vi "Version_4.9_8_on-chip_valves_for25ulSyringe_withModfied_Plunging.vi"() -> ()   [LabVIEW 2020] (continued)
                            n2712 = local write "Valve V2 Open"(FALSE ("Valve V2 Open")) -> ()
                            n2713 = local write "Valve V3 Open"(FALSE ("Valve V3 Open")) -> ()
                            n2714 = local write "Valve V4 Open"(TRUE ("Valve V4 Open")) -> ()
                            n2715 = call "PortChanger_Valve (SubVI).vi"("Port Number"=w3158, "VISA Refnum in"=w3159) -> ()  [unwired: 10 in]
                            n2716 = local write "Valve V5 Open"(TRUE ("Valve V5 Open")) -> ()
                            n2717 = local write "Valve V6 Open"(TRUE ("Valve V6 Open")) -> ()
                            n2718 = local write "Valve V7 Open"(FALSE ("Valve V7 Open")) -> ()
                          }
                          frame #3 {
                            n2719 = local read "Apparent Volume\nof Syringe"() -> (w3164:dbl)
                            n2720 = local read "Sample Volume \nto be Pumped"() -> (w3167:dbl)
                            n2721 = Quotient & Remainder(x=w3167, y=w3164) -> (x-y*floor(x/y)=w3165:dbl, floor(x/y)=w3166:dbl)
                            n2722 = for {
                              N: w3166 -> [_]
                              n2723 = stacked-sequence {
                                frame #0 {
                                n2724 = local read "Sample PickUp \nFlow Rate (ul/min)"() -> (w3170:dbl)
                                n2725 = local read "Sample Pumping\nResolution"() -> (w3169:T2)
                                n2726 = local read "VISA Refnum in\nfor Pump"() -> (w3172:refnum<visa-resource-name>)
                                n2727 = local read "Apparent Volume\nof Syringe"() -> (w3168:dbl)
                                n2728 = local read "Volume of Syringe"() -> (w3171:dbl)
                                n2729 = call "RPickUp(SubVI).vi"("Volume to be picked up"=w3168, "Volume of Syringe"=w3171, "Resolution of PickUP"=w3169, "PickUp Flow Rate (ul/min)"=w3170, "VISA Refnum in"=w3172) -> ()  [unwired: 6 in, 1 out]
                                }
                                frame #1 {
                                n2730 = local read "Stopper that ends \nthe main loops"() -> (w3173:bool)
                                n2731 = local read "VISA Refnum in\nfor Pump"() -> (w3174:refnum<visa-resource-name>)
                                n2732 = case shown="True" w3173 {
                                frame False {
                                }
                                frame True {
                                n2733 = local read "VISA Refnum in\nfor Pump"() -> (w3175:refnum<visa-resource-name>)
                                n2734 = call "HardStopCurrentProcess (SubVI).vi"("VISA Refnum in"=w3175) -> ()  [unwired: 11 in]
                                }
                                }
                                n2735 = call "ProcessCompletionWaiter (SubVI).vi"("VISA Refnum in"=w3174) -> ()  [unwired: 11 in]
                                }
                                frame #2 {
                                # "Reads the initial Plunger Position for computing the volume dispensed"
                                n2736 = local read "VISA Refnum in\nfor Pump"() -> (w3177:refnum<visa-resource-name>)
                                n2737 = call "AbsolutePlungerPosition (SubVI).vi"("VISA Refnum in"=w3177) -> ("Plunger Position"=w3176:i32)  [unwired: 10 in]
                                n2738 = local write "Initial Plunger Position"(w3176) -> ()
                                }
                                frame #3 {
                                # "Switch to Port-2"
                                # "Port-2 of the pump is conncted to column-1 of chip"
                                n2739 = local read "VISA Refnum in\nfor Pump"() -> (w3179:refnum<visa-resource-name>)
                                n2740 = call "PortChanger (SubVI).vi"("Port Number"="10", "VISA Refnum in"=w3179) -> ()  [unwired: 10 in]
                                }
                                frame #4 {
                                n2741 = local read "Stopper that ends \nthe main loops"() -> (w3180:bool)
                                n2742 = local read "VISA Refnum in\nfor Pump"() -> (w3181:refnum<visa-resource-name>)
                                n2743 = case shown="True" w3180 {
                                frame False {
                                }
                                frame True {
                                n2744 = local read "VISA Refnum in\nfor Pump"() -> (w3182:refnum<visa-resource-name>)
                                n2745 = call "HardStopCurrentProcess (SubVI).vi"("VISA Refnum in"=w3182) -> ()  [unwired: 11 in]
                                }
                                }
                                n2746 = call "ProcessCompletionWaiter (SubVI).vi"("VISA Refnum in"=w3181) -> ()  [unwired: 11 in]
                                }
                                frame #5 {
                                # "Keeps the AMF valve after column-1 open and valve after column-2 closed"
                                n2747 = local read "Sample Dispense\nFlow Rate (ul/min)"() -> (w3186:dbl)
                                n2748 = local read "Sample Pumping\nResolution"() -> (w3185:T2)
                                n2749 = local read "VISA Refnum in\nfor Pump"() -> (w3188:refnum<visa-resource-name>)
                                n2750 = local write "Pause Data Collection"(FALSE ("Pause Data Collection")) -> ()
                                n2751 = local read "Volume of Syringe"() -> (w3187:dbl)
                                n2752 = call "GoToAbsolutePosition(SubVI).vi"("Absolute Volume Position in Syringe (in ul)"=0.0 ("Volume to be Dispensed"), "Volume of Syringe"=w3187, "Resolution of Pumping"=w3185, "Flow Rate (ul/min)"=w3186, "VISA Refnum in"=w3188) -> ()  [unwired: 6 in, 1 out]
                                }
                                frame #6 {
                                n2753 = local read "Sample Pumping\nResolution"() -> (w3190:T2)
                                n2754 = local read "VISA Refnum in\nfor Pump"() -> (w3192:refnum<visa-resource-name>)
                                n2755 = local read "Initial Plunger Position"() -> (w3191:dbl)
                                n2756 = local read "Volume of Syringe"() -> (w3189:dbl)
                                n2757 = while {
                                tunnel: w3191 -> [w3199]
                                tunnel: w3192 -> [w3198]
                                tunnel: w3190 -> [w3197]
                                tunnel: w3189 -> [w3196]
                                stop <- w3194 stop-if-true
                                n2758 = stacked-sequence {
                                tunnel: w3199 -> [w3206 _]
                                tunnel: w3198 -> [w3205 w3226]
                                tunnel: w3197 -> [w3204 _]
                                tunnel: w3196 -> [w3203 _]
                                tunnel: [_ w3224] -> w3194
                                frame #0 {
                                n2759 = call "AbsolutePlungerPosition (SubVI).vi"("VISA Refnum in"=w3205) -> ("Plunger Position"=w3202:i32)  [unwired: 10 in]
                                n2760 = case shown="\"Standard Pumping\", Default" w3204 {
                                tunnel: w3206 -> [w3211 w3220]
                                tunnel: w3202 -> [w3212 w3219]
                                tunnel: [w3210 w3217] -> w3201
                                tunnel: w3203 -> [w3209 w3218]
                                frame "Standard Pumping", Default {
                                n2761 = Subtract(x=w3211, y=w3212) -> (x-y=w3208:dbl)
                                n2762 = Absolute Value(x=w3208) -> (abs(x)=w3207:dbl)
                                n2763 = Multiply(x=w3207, y=w3209) -> (x*y=w3214:dbl)
                                n2764 = Divide(x=w3214, y=3000.0) -> (x/y=w3210:dbl)
                                }
                                frame "High Resolution Pumping" {
                                n2765 = Subtract(x=w3220, y=w3219) -> (x-y=w3216:dbl)
                                n2766 = Absolute Value(x=w3216) -> (abs(x)=w3215:dbl)
                                n2767 = Multiply(x=w3215, y=w3218) -> (x*y=w3222:dbl)
                                n2768 = Divide(x=w3222, y=24000.0) -> (x/y=w3217:dbl)
                                }
                                }
                                n2769 = local write "Volume being Injected \nin this process"(w3201) -> ()
                                }
                                frame #1 {
                                n2770 = call "LSPOneStatus (SubVI).vi"("VISA Refnum in"=w3226) -> ("read buffer"=w3228:string)  [unwired: 10 in]
                                n2771 = call <vilib>:"Trim Whitespace.vi"("string"=w3228) -> ("trimmed string"=w3227:string)  [unwired: 1 in]
                                n2772 = local read "Stopper that ends \nthe main loops"() -> (w3223:bool)
                                n2773 = Equal?(x=w3227, y="/0`\u0003") -> (x = y?=w3225:bool)
                                n2774 = Or(x=w3225, y=w3223) -> (x .or. y?=w3224:bool)
                                }
                                }
                                n2775 = Wait (ms)(milliseconds to wait=u32 100) -> ()  [unwired: 1 out]
                                n2776 = local read "Stopper that ends \nthe main loops"() -> (w3193:bool)
                                n2777 = case shown="True" w3193 {
                                frame False {
                                }
                                frame True {
                                n2778 = local read "VISA Refnum in\nfor Pump"() -> (w3200:refnum<visa-resource-name>)
                                n2779 = call "HardStopCurrentProcess (SubVI).vi"("VISA Refnum in"=w3200) -> ()  [unwired: 11 in]
                                }
                                }
                                }
                                }
                                frame #7 {
                                # "Chnage the pump port back to Sample"
                                n2780 = local read "VISA Refnum in\nfor Pump"() -> (w3231:refnum<visa-resource-name>)
                                n2781 = local read "Port for \nSample"() -> (w3230:string)
                                n2782 = local write "Pause Data Collection"(TRUE ("Pause Data Collection")) -> ()
                                n2783 = Wait (ms)(milliseconds to wait=u32 500) -> ()  [unwired: 1 out]
                                n2784 = call "PortChanger (SubVI).vi"("Port Number"=w3230, "VISA Refnum in"=w3231) -> ()  [unwired: 10 in]
                                }
                                frame #8 {
                                n2785 = local read "VISA Refnum in\nfor Pump"() -> (w3234:refnum<visa-resource-name>)
                                n2786 = local write "Volume being Injected \nin this process"(0.0 ("Volume being Injected \nin this process")) -> ()
                                n2787 = call "ProcessCompletionWaiter (SubVI).vi"("VISA Refnum in"=w3234) -> ()  [unwired: 11 in]
                                }
                              }
                            }
                            n2788 = local write "Reminder of the \nVolume to be \nPumped"(w3165) -> ()
                          }
                          frame #4 {
                            n2789 = stacked-sequence {
                              frame #0 {
                                n2790 = local read "Sample PickUp \nFlow Rate (ul/min)"() -> (w3238:dbl)
                                n2791 = local read "Sample Pumping\nResolution"() -> (w3237:T2)
                                n2792 = local read "VISA Refnum in\nfor Pump"() -> (w3240:refnum<visa-resource-name>)
                                n2793 = local read "Reminder of the \nVolume to be \nPumped"() -> (w3236:dbl)
                                n2794 = local read "Volume of Syringe"() -> (w3239:dbl)
                                n2795 = call "RPickUp(SubVI).vi"("Volume to be picked up"=w3236, "Volume of Syringe"=w3239, "Resolution of PickUP"=w3237, "PickUp Flow Rate (ul/min)"=w3238, "VISA Refnum in"=w3240) -> ()  [unwired: 6 in, 1 out]
                              }
                              frame #1 {
                                n2796 = local read "Stopper that ends \nthe main loops"() -> (w3241:bool)
                                n2797 = local read "VISA Refnum in\nfor Pump"() -> (w3242:refnum<visa-resource-name>)
                                n2798 = case shown="True" w3241 {
                                frame False {
                                }
                                frame True {
                                n2799 = local read "VISA Refnum in\nfor Pump"() -> (w3243:refnum<visa-resource-name>)
                                n2800 = call "HardStopCurrentProcess (SubVI).vi"("VISA Refnum in"=w3243) -> ()  [unwired: 11 in]
                                }
                                }
                                n2801 = call "ProcessCompletionWaiter (SubVI).vi"("VISA Refnum in"=w3242) -> ()  [unwired: 11 in]
                              }
                              frame #2 {
                                # "Reads the initial Plunger Position for computing the volume dispensed"
                                n2802 = local read "VISA Refnum in\nfor Pump"() -> (w3245:refnum<visa-resource-name>)
                                n2803 = call "AbsolutePlungerPosition (SubVI).vi"("VISA Refnum in"=w3245) -> ("Plunger Position"=w3244:i32)  [unwired: 10 in]
                                n2804 = local write "Initial Plunger Position"(w3244) -> ()
                              }
                              frame #3 {
                                # "Switch to Port-2"
                                # "Port-2 of the pump is conncted to column-1 of chip"
                                n2805 = local read "VISA Refnum in\nfor Pump"() -> (w3247:refnum<visa-resource-name>)
                                n2806 = call "PortChanger (SubVI).vi"("Port Number"="10", "VISA Refnum in"=w3247) -> ()  [unwired: 10 in]
                              }
                              frame #4 {
                                n2807 = local read "Stopper that ends \nthe main loops"() -> (w3248:bool)
                                n2808 = local read "VISA Refnum in\nfor Pump"() -> (w3249:refnum<visa-resource-name>)
                                n2809 = case shown="True" w3248 {
                                frame False {
                                }
                                frame True {
                                n2810 = local read "VISA Refnum in\nfor Pump"() -> (w3250:refnum<visa-resource-name>)
                                n2811 = call "HardStopCurrentProcess (SubVI).vi"("VISA Refnum in"=w3250) -> ()  [unwired: 11 in]
                                }
                                }
                                n2812 = call "ProcessCompletionWaiter (SubVI).vi"("VISA Refnum in"=w3249) -> ()  [unwired: 11 in]
                              }
                              frame #5 {
                                # "Keeps the AMF valve after column-1 open and valve after column-2 closed"
                                n2813 = local read "Sample Dispense\nFlow Rate (ul/min)"() -> (w3254:dbl)
                                n2814 = local read "Sample Pumping\nResolution"() -> (w3253:T2)
                                n2815 = local read "VISA Refnum in\nfor Pump"() -> (w3256:refnum<visa-resource-name>)
                                n2816 = local write "Pause Data Collection"(FALSE ("Pause Data Collection")) -> ()
                                n2817 = local read "Volume of Syringe"() -> (w3255:dbl)
                                n2818 = call "GoToAbsolutePosition(SubVI).vi"("Absolute Volume Position in Syringe (in ul)"=0.0 ("Volume to be Dispensed"), "Volume of Syringe"=w3255, "Resolution of Pumping"=w3253, "Flow Rate (ul/min)"=w3254, "VISA Refnum in"=w3256) -> ()  [unwired: 6 in, 1 out]
                              }
                              frame #6 {
                                n2819 = local read "Sample Pumping\nResolution"() -> (w3258:T2)
                                n2820 = local read "VISA Refnum in\nfor Pump"() -> (w3260:refnum<visa-resource-name>)
                                n2821 = local read "Initial Plunger Position"() -> (w3259:dbl)
                                n2822 = local read "Volume of Syringe"() -> (w3257:dbl)
                                n2823 = while {
                                tunnel: w3259 -> [w3267]
                                tunnel: w3260 -> [w3266]
                                tunnel: w3258 -> [w3265]
                                tunnel: w3257 -> [w3264]
                                stop <- w3262 stop-if-true
                                n2824 = stacked-sequence {
                                tunnel: w3267 -> [w3274 _]
                                tunnel: w3266 -> [w3273 w3294]
                                tunnel: w3265 -> [w3272 _]
                                tunnel: w3264 -> [w3271 _]
                                tunnel: [_ w3292] -> w3262
                                frame #0 {
                                n2825 = call "AbsolutePlungerPosition (SubVI).vi"("VISA Refnum in"=w3273) -> ("Plunger Position"=w3270:i32)  [unwired: 10 in]
                                n2826 = case shown="\"Standard Pumping\", Default" w3272 {
                                tunnel: w3274 -> [w3279 w3288]
                                tunnel: w3270 -> [w3280 w3287]
                                tunnel: [w3278 w3285] -> w3269
                                tunnel: w3271 -> [w3277 w3286]
                                frame "Standard Pumping", Default {
                                n2827 = Subtract(x=w3279, y=w3280) -> (x-y=w3276:dbl)
                                n2828 = Absolute Value(x=w3276) -> (abs(x)=w3275:dbl)
                                n2829 = Multiply(x=w3275, y=w3277) -> (x*y=w3282:dbl)
                                n2830 = Divide(x=w3282, y=3000.0) -> (x/y=w3278:dbl)
                                }
                                frame "High Resolution Pumping" {
                                n2831 = Subtract(x=w3288, y=w3287) -> (x-y=w3284:dbl)
                                n2832 = Absolute Value(x=w3284) -> (abs(x)=w3283:dbl)
                                n2833 = Multiply(x=w3283, y=w3286) -> (x*y=w3290:dbl)
                                n2834 = Divide(x=w3290, y=24000.0) -> (x/y=w3285:dbl)
                                }
                                }
                                n2835 = local write "Volume being Injected \nin this process"(w3269) -> ()
                                }
                                frame #1 {
                                n2836 = call "LSPOneStatus (SubVI).vi"("VISA Refnum in"=w3294) -> ("read buffer"=w3296:string)  [unwired: 10 in]
                                n2837 = call <vilib>:"Trim Whitespace.vi"("string"=w3296) -> ("trimmed string"=w3295:string)  [unwired: 1 in]
                                n2838 = local read "Stopper that ends \nthe main loops"() -> (w3291:bool)
                                n2839 = Equal?(x=w3295, y="/0`\u0003") -> (x = y?=w3293:bool)
                                n2840 = Or(x=w3293, y=w3291) -> (x .or. y?=w3292:bool)
                                }
                                }
                                n2841 = Wait (ms)(milliseconds to wait=u32 100) -> ()  [unwired: 1 out]
                                n2842 = local read "Stopper that ends \nthe main loops"() -> (w3261:bool)
                                n2843 = case shown="True" w3261 {
                                frame False {
                                }
                                frame True {
                                n2844 = local read "VISA Refnum in\nfor Pump"() -> (w3268:refnum<visa-resource-name>)
                                n2845 = call "HardStopCurrentProcess (SubVI).vi"("VISA Refnum in"=w3268) -> ()  [unwired: 11 in]
                                }
                                }
                                }
                              }
                              frame #7 {
                                n2846 = local write "Pause Data Collection"(TRUE ("Pause Data Collection")) -> ()
                                n2847 = Wait (ms)(milliseconds to wait=u32 500) -> ()  [unwired: 1 out]
                              }
                              frame #8 {
                                n2848 = local write "Volume being Injected \nin this process"(0.0 ("Volume being Injected \nin this process")) -> ()
                              }
                            }
                          }
                        }
                        n2849 = local write "Equilibriating \nColumn-2"(FALSE ("Equilibriating \nColumn-2")) -> ()
                        n2850 = local write "Affinity On"(TRUE ("Affinity On")) -> ()
                        n2851 = local write "Sample pumping \ninto Column-1"(TRUE ("Sample pumping \ninto Column-1")) -> ()
                      }
                      frame #2 {
                        # "Wash Column-1 with Buffer-A2"
                        n2852 = stacked-sequence {
                          frame #0 {
                            # "Switch to Port-4/6"
                            # "Port-4/6 of pump is connected to Buffer-A2"
                            n2853 = local read "VISA Refnum in\nfor Pump"() -> (w3304:refnum<visa-resource-name>)
                            n2854 = local read "Port for \nA2-Wash"() -> (w3303:string)
                            n2855 = call "PortChanger (SubVI).vi"("Port Number"=w3303, "VISA Refnum in"=w3304) -> ()  [unwired: 10 in]
                          }
                          frame #1 {
                            n2856 = local read "VISA Refnum in\nfor Pump"() -> (w3305:refnum<visa-resource-name>)
                            n2857 = call "ProcessCompletionWaiter (SubVI).vi"("VISA Refnum in"=w3305) -> ()  [unwired: 11 in]
                          }
                          frame #2 {
                            n2858 = local read "VISA Refnum in\nfor Valve"() -> (w3309:refnum<visa-resource-name>)
                            n2859 = local read "External Valve \nOPEN"() -> (w3310:string)
                            n2860 = local write "Valve V3 Open"(FALSE ("Valve V3 Open")) -> ()
                            n2861 = local write "Valve V4 Open"(FALSE ("Valve V4 Open")) -> ()
                            n2862 = local write "Valve V1 Open"(TRUE ("Valve V1 Open")) -> ()
                            n2863 = local write "Valve V2 Open"(TRUE ("Valve V2 Open")) -> ()
                            n2864 = call "PortChanger_Valve (SubVI).vi"("Port Number"=w3310, "VISA Refnum in"=w3309) -> ()  [unwired: 10 in]
                            n2865 = local write "Valve V5 Open"(FALSE ("Valve V5 Open")) -> ()
                            n2866 = local write "Valve V6 Open"(FALSE ("Valve V6 Open")) -> ()
                            n2867 = local write "Valve V7 Open"(FALSE ("Valve V7 Open")) -> ()
                          }
                          frame #3 {
                            n2868 = local read "Buffer-A2 Volume \nto be Pumped"() -> (w3318:dbl)
                            n2869 = local read "Apparent Volume\nof Syringe"() -> (w3315:dbl)
                            n2870 = Quotient & Remainder(x=w3318, y=w3315) -> (x-y*floor(x/y)=w3316:dbl, floor(x/y)=w3317:dbl)
                            n2871 = for {
                              N: w3317 -> [_]
                              n2872 = stacked-sequence {
                                frame #0 {
                                n2873 = local read "Buffer-A2 PickUp \nFlow Rate (ul/min)"() -> (w3321:dbl)
                                n2874 = local read "Buffer-A2 Pumping\nResolution"() -> (w3320:T2)
                                n2875 = local read "VISA Refnum in\nfor Pump"() -> (w3323:refnum<visa-resource-name>)
                                n2876 = local read "Apparent Volume\nof Syringe"() -> (w3319:dbl)
                                n2877 = local read "Volume of Syringe"() -> (w3322:dbl)
                                n2878 = call "RPickUp(SubVI).vi"("Volume to be picked up"=w3319, "Volume of Syringe"=w3322, "Resolution of PickUP"=w3320, "PickUp Flow Rate (ul/min)"=w3321, "VISA Refnum in"=w3323) -> ()  [unwired: 6 in, 1 out]
                                }
                                frame #1 {
                                n2879 = local read "Stopper that ends \nthe main loops"() -> (w3324:bool)
                                n2880 = local read "VISA Refnum in\nfor Pump"() -> (w3325:refnum<visa-resource-name>)
                                n2881 = case shown="True" w3324 {
                                frame False {
                                }
                                frame True {
                                n2882 = local read "VISA Refnum in\nfor Pump"() -> (w3326:refnum<visa-resource-name>)
                                n2883 = call "HardStopCurrentProcess (SubVI).vi"("VISA Refnum in"=w3326) -> ()  [unwired: 11 in]
                                }
                                }
                                n2884 = call "ProcessCompletionWaiter (SubVI).vi"("VISA Refnum in"=w3325) -> ()  [unwired: 11 in]
                                }
                                frame #2 {
                                # "Reads the initial Plunger Position for computing the volume dispensed"
                                n2885 = local read "VISA Refnum in\nfor Pump"() -> (w3328:refnum<visa-resource-name>)
                                n2886 = call "AbsolutePlungerPosition (SubVI).vi"("VISA Refnum in"=w3328) -> ("Plunger Position"=w3327:i32)  [unwired: 10 in]
                                n2887 = local write "Initial Plunger Position"(w3327) -> ()
                                }
                                frame #3 {
                                # "Switch to Port-2"
                                # "Port-2 of the pump is conncted to column-1 of chip"
                                n2888 = local read "VISA Refnum in\nfor Pump"() -> (w3330:refnum<visa-resource-name>)
                                n2889 = call "PortChanger (SubVI).vi"("Port Number"="2", "VISA Refnum in"=w3330) -> ()  [unwired: 10 in]
                                }
                                frame #4 {
                                n2890 = local read "Stopper that ends \nthe main loops"() -> (w3331:bool)
                                n2891 = local read "VISA Refnum in\nfor Pump"() -> (w3332:refnum<visa-resource-name>)
                                n2892 = case shown="True" w3331 {
                                frame False {
                                }
                                frame True {
                                n2893 = local read "VISA Refnum in\nfor Pump"() -> (w3333:refnum<visa-resource-name>)
                                n2894 = call "HardStopCurrentProcess (SubVI).vi"("VISA Refnum in"=w3333) -> ()  [unwired: 11 in]
                                }
                                }
                                n2895 = call "ProcessCompletionWaiter (SubVI).vi"("VISA Refnum in"=w3332) -> ()  [unwired: 11 in]
                                }
                                frame #5 {
                                # "Keeps the AMF valve after column-1 open and valve after column-2 closed"
                                n2896 = local read "Buffer-A2 Dispense\nFlow Rate (ul/min)"() -> (w3337:dbl)
                                n2897 = local read "Buffer-A2 Pumping\nResolution"() -> (w3336:T2)
                                n2898 = local read "VISA Refnum in\nfor Pump"() -> (w3339:refnum<visa-resource-name>)
                                n2899 = local write "Pause Data Collection"(FALSE ("Pause Data Collection")) -> ()
                                n2900 = local read "Volume of Syringe"() -> (w3338:dbl)
                                n2901 = call "GoToAbsolutePosition(SubVI).vi"("Absolute Volume Position in Syringe (in ul)"=0.0 ("Volume to be Dispensed"), "Volume of Syringe"=w3338, "Resolution of Pumping"=w3336, "Flow Rate (ul/min)"=w3337, "VISA Refnum in"=w3339) -> ()  [unwired: 6 in, 1 out]
                                }
                                frame #6 {
                                n2902 = local read "Buffer-A2 Pumping\nResolution"() -> (w3341:T2)
                                n2903 = local read "VISA Refnum in\nfor Pump"() -> (w3343:refnum<visa-resource-name>)
                                n2904 = local read "Initial Plunger Position"() -> (w3342:dbl)
                                n2905 = local read "Volume of Syringe"() -> (w3340:dbl)
                                n2906 = while {
                                tunnel: w3342 -> [w3350]
                                tunnel: w3343 -> [w3349]
                                tunnel: w3341 -> [w3348]
                                tunnel: w3340 -> [w3347]
                                stop <- w3345 stop-if-true
                                n2907 = stacked-sequence {
                                tunnel: w3350 -> [w3357 _]
                                tunnel: w3349 -> [w3356 w3377]
                                tunnel: w3348 -> [w3355 _]
                                tunnel: w3347 -> [w3354 _]
                                tunnel: [_ w3375] -> w3345
                                frame #0 {
                                n2908 = call "AbsolutePlungerPosition (SubVI).vi"("VISA Refnum in"=w3356) -> ("Plunger Position"=w3353:i32)  [unwired: 10 in]
                                n2909 = case shown="\"Standard Pumping\", Default" w3355 {
                                tunnel: w3357 -> [w3362 w3371]
                                tunnel: w3353 -> [w3363 w3370]
                                tunnel: [w3361 w3368] -> w3352
                                tunnel: w3354 -> [w3360 w3369]
                                frame "Standard Pumping", Default {
                                n2910 = Subtract(x=w3362, y=w3363) -> (x-y=w3359:dbl)
                                n2911 = Absolute Value(x=w3359) -> (abs(x)=w3358:dbl)
                                n2912 = Multiply(x=w3358, y=w3360) -> (x*y=w3365:dbl)
                                n2913 = Divide(x=w3365, y=3000.0) -> (x/y=w3361:dbl)
                                }
                                frame "High Resolution Pumping" {
                                n2914 = Subtract(x=w3371, y=w3370) -> (x-y=w3367:dbl)
                                n2915 = Absolute Value(x=w3367) -> (abs(x)=w3366:dbl)
                                n2916 = Multiply(x=w3366, y=w3369) -> (x*y=w3373:dbl)
                                n2917 = Divide(x=w3373, y=24000.0) -> (x/y=w3368:dbl)
                                }
                                }
                                n2918 = local write "Volume being Injected \nin this process"(w3352) -> ()
                                }
                                frame #1 {
                                n2919 = call "LSPOneStatus (SubVI).vi"("VISA Refnum in"=w3377) -> ("read buffer"=w3379:string)  [unwired: 10 in]
                                n2920 = call <vilib>:"Trim Whitespace.vi"("string"=w3379) -> ("trimmed string"=w3378:string)  [unwired: 1 in]
                                n2921 = local read "Stopper that ends \nthe main loops"() -> (w3374:bool)
                                n2922 = Equal?(x=w3378, y="/0`\u0003") -> (x = y?=w3376:bool)
                                n2923 = Or(x=w3376, y=w3374) -> (x .or. y?=w3375:bool)
                                }
                                }
                                n2924 = Wait (ms)(milliseconds to wait=u32 100) -> ()  [unwired: 1 out]
                                n2925 = local read "Stopper that ends \nthe main loops"() -> (w3344:bool)
                                n2926 = case shown="True" w3344 {
                                frame False {
                                }
                                frame True {
                                n2927 = local read "VISA Refnum in\nfor Pump"() -> (w3351:refnum<visa-resource-name>)
                                n2928 = call "HardStopCurrentProcess (SubVI).vi"("VISA Refnum in"=w3351) -> ()  [unwired: 11 in]
                                }
                                }
                                }
                                }
                                frame #7 {
                                # "Change the port back to Buffer-A2"
                                n2929 = local read "VISA Refnum in\nfor Pump"() -> (w3382:refnum<visa-resource-name>)
                                n2930 = local read "Port for \nA2-Wash"() -> (w3381:string)
                                n2931 = local write "Pause Data Collection"(TRUE ("Pause Data Collection")) -> ()
                                n2932 = Wait (ms)(milliseconds to wait=u32 500) -> ()  [unwired: 1 out]
                                n2933 = call "PortChanger (SubVI).vi"("Port Number"=w3381, "VISA Refnum in"=w3382) -> ()  [unwired: 10 in]
                                }
                                frame #8 {
                                n2934 = local read "VISA Refnum in\nfor Pump"() -> (w3385:refnum<visa-resource-name>)
                                n2935 = local write "Volume being Injected \nin this process"(0.0 ("Volume being Injected \nin this process")) -> ()
                                n2936 = call "ProcessCompletionWaiter (SubVI).vi"("VISA Refnum in"=w3385) -> ()  [unwired: 11 in]
                                }
                              }
                            }
                            n2937 = local write "Reminder of the \nVolume to be \nPumped"(w3316) -> ()
                          }
                          frame #4 {
                            n2938 = stacked-sequence {
                              frame #0 {
                                n2939 = local read "Buffer-A2 PickUp \nFlow Rate (ul/min)"() -> (w3389:dbl)
                                n2940 = local read "Buffer-A2 Pumping\nResolution"() -> (w3388:T2)
                                n2941 = local read "VISA Refnum in\nfor Pump"() -> (w3391:refnum<visa-resource-name>)
                                n2942 = local read "Reminder of the \nVolume to be \nPumped"() -> (w3387:dbl)
                                n2943 = local read "Volume of Syringe"() -> (w3390:dbl)
                                n2944 = call "RPickUp(SubVI).vi"("Volume to be picked up"=w3387, "Volume of Syringe"=w3390, "Resolution of PickUP"=w3388, "PickUp Flow Rate (ul/min)"=w3389, "VISA Refnum in"=w3391) -> ()  [unwired: 6 in, 1 out]
                              }
                              frame #1 {
                                n2945 = local read "Stopper that ends \nthe main loops"() -> (w3392:bool)
                                n2946 = local read "VISA Refnum in\nfor Pump"() -> (w3393:refnum<visa-resource-name>)
                                n2947 = case shown="True" w3392 {
                                frame False {
                                }
                                frame True {
                                n2948 = local read "VISA Refnum in\nfor Pump"() -> (w3394:refnum<visa-resource-name>)
                                n2949 = call "HardStopCurrentProcess (SubVI).vi"("VISA Refnum in"=w3394) -> ()  [unwired: 11 in]
                                }
                                }
                                n2950 = call "ProcessCompletionWaiter (SubVI).vi"("VISA Refnum in"=w3393) -> ()  [unwired: 11 in]
                              }
                              frame #2 {
                                # "Reads the initial Plunger Position for computing the volume dispensed"
                                n2951 = local read "VISA Refnum in\nfor Pump"() -> (w3396:refnum<visa-resource-name>)
                                n2952 = call "AbsolutePlungerPosition (SubVI).vi"("VISA Refnum in"=w3396) -> ("Plunger Position"=w3395:i32)  [unwired: 10 in]
                                n2953 = local write "Initial Plunger Position"(w3395) -> ()
                              }
                              frame #3 {
                                # "Switch to Port-2"
                                # "Port-2 of the pump is conncted to column-1 of chip"
                                n2954 = local read "VISA Refnum in\nfor Pump"() -> (w3398:refnum<visa-resource-name>)
                                n2955 = call "PortChanger (SubVI).vi"("Port Number"="2", "VISA Refnum in"=w3398) -> ()  [unwired: 10 in]
                              }
                              frame #4 {
                                n2956 = local read "Stopper that ends \nthe main loops"() -> (w3399:bool)
                                n2957 = local read "VISA Refnum in\nfor Pump"() -> (w3400:refnum<visa-resource-name>)
                                n2958 = case shown="True" w3399 {
                                frame False {
                                }
                                frame True {
                                n2959 = local read "VISA Refnum in\nfor Pump"() -> (w3401:refnum<visa-resource-name>)
                                n2960 = call "HardStopCurrentProcess (SubVI).vi"("VISA Refnum in"=w3401) -> ()  [unwired: 11 in]
                                }
                                }
                                n2961 = call "ProcessCompletionWaiter (SubVI).vi"("VISA Refnum in"=w3400) -> ()  [unwired: 11 in]
                              }
                              frame #5 {
                                # "Keeps the AMF valve after column-1 open and valve after column-2 closed"
                                n2962 = local read "Buffer-A2 Dispense\nFlow Rate (ul/min)"() -> (w3405:dbl)
                                n2963 = local read "Buffer-A2 Pumping\nResolution"() -> (w3404:T2)
                                n2964 = local read "VISA Refnum in\nfor Pump"() -> (w3407:refnum<visa-resource-name>)
                                n2965 = local write "Pause Data Collection"(FALSE ("Pause Data Collection")) -> ()
                                n2966 = local read "Volume of Syringe"() -> (w3406:dbl)
                                n2967 = call "GoToAbsolutePosition(SubVI).vi"("Absolute Volume Position in Syringe (in ul)"=0.0 ("Volume to be Dispensed"), "Volume of Syringe"=w3406, "Resolution of Pumping"=w3404, "Flow Rate (ul/min)"=w3405, "VISA Refnum in"=w3407) -> ()  [unwired: 6 in, 1 out]
                              }
                              frame #6 {
                                n2968 = local read "Buffer-A2 Pumping\nResolution"() -> (w3409:T2)
                                n2969 = local read "VISA Refnum in\nfor Pump"() -> (w3411:refnum<visa-resource-name>)
                                n2970 = local read "Initial Plunger Position"() -> (w3410:dbl)
                                n2971 = local read "Volume of Syringe"() -> (w3408:dbl)
                                n2972 = while {
                                tunnel: w3410 -> [w3418]
                                tunnel: w3411 -> [w3417]
                                tunnel: w3409 -> [w3416]
                                tunnel: w3408 -> [w3415]
                                stop <- w3413 stop-if-true
                                n2973 = stacked-sequence {
                                tunnel: w3418 -> [w3425 _]
                                tunnel: w3417 -> [w3424 w3445]
                                tunnel: w3416 -> [w3423 _]
                                tunnel: w3415 -> [w3422 _]
                                tunnel: [_ w3443] -> w3413
                                frame #0 {
                                n2974 = call "AbsolutePlungerPosition (SubVI).vi"("VISA Refnum in"=w3424) -> ("Plunger Position"=w3421:i32)  [unwired: 10 in]
                                n2975 = case shown="\"Standard Pumping\", Default" w3423 {
                                tunnel: w3425 -> [w3430 w3439]
                                tunnel: w3421 -> [w3431 w3438]
                                tunnel: [w3429 w3436] -> w3420
                                tunnel: w3422 -> [w3428 w3437]
                                frame "Standard Pumping", Default {
                                n2976 = Subtract(x=w3430, y=w3431) -> (x-y=w3427:dbl)
                                n2977 = Absolute Value(x=w3427) -> (abs(x)=w3426:dbl)
                                n2978 = Multiply(x=w3426, y=w3428) -> (x*y=w3433:dbl)
                                n2979 = Divide(x=w3433, y=3000.0) -> (x/y=w3429:dbl)
                                }
                                frame "High Resolution Pumping" {
                                n2980 = Subtract(x=w3439, y=w3438) -> (x-y=w3435:dbl)
                                n2981 = Absolute Value(x=w3435) -> (abs(x)=w3434:dbl)
                                n2982 = Multiply(x=w3434, y=w3437) -> (x*y=w3441:dbl)
                                n2983 = Divide(x=w3441, y=24000.0) -> (x/y=w3436:dbl)
                                }
                                }
                                n2984 = local write "Volume being Injected \nin this process"(w3420) -> ()
                                }
                                frame #1 {
                                n2985 = call "LSPOneStatus (SubVI).vi"("VISA Refnum in"=w3445) -> ("read buffer"=w3447:string)  [unwired: 10 in]
                                n2986 = call <vilib>:"Trim Whitespace.vi"("string"=w3447) -> ("trimmed string"=w3446:string)  [unwired: 1 in]
                                n2987 = local read "Stopper that ends \nthe main loops"() -> (w3442:bool)
                                n2988 = Equal?(x=w3446, y="/0`\u0003") -> (x = y?=w3444:bool)
                                n2989 = Or(x=w3444, y=w3442) -> (x .or. y?=w3443:bool)
                                }
                                }
                                n2990 = Wait (ms)(milliseconds to wait=u32 100) -> ()  [unwired: 1 out]
                                n2991 = local read "Stopper that ends \nthe main loops"() -> (w3412:bool)
                                n2992 = case shown="True" w3412 {
                                frame False {
                                }
                                frame True {
                                n2993 = local read "VISA Refnum in\nfor Pump"() -> (w3419:refnum<visa-resource-name>)
                                n2994 = call "HardStopCurrentProcess (SubVI).vi"("VISA Refnum in"=w3419) -> ()  [unwired: 11 in]
                                }
                                }
                                }
                              }
                              frame #7 {
                                n2995 = local write "Pause Data Collection"(TRUE ("Pause Data Collection")) -> ()
                                n2996 = Wait (ms)(milliseconds to wait=u32 500) -> ()  [unwired: 1 out]
                              }
                              frame #8 {
                                n2997 = local write "Volume being Injected \nin this process"(0.0 ("Volume being Injected \nin this process")) -> ()
                                n2998 = local write "Start the Process"(FALSE ("Start the Process")) -> ()
                              }
                            }
                          }
                        }
                        n2999 = local write "Sample pumping \ninto Column-1"(FALSE ("Sample pumping \ninto Column-1")) -> ()
                        n3000 = local write "Washing Column-1"(TRUE ("Washing Column-1")) -> ()
                      }
                      frame #3 {
                        # "Connecting Buffer-C with port-5, cleaning the tubing with Buffer-C1, and washing the Column-2 to get rid of spill out from wash steps of column-1"
                        n3001 = stacked-sequence {
                          frame #0 {
                            # "Switch to Port-5"
                            # "Port-5 of pump is connected to Buffer-C1"
                            n3002 = local read "VISA Refnum in\nfor Pump"() -> (w3456:refnum<visa-resource-name>)
                            n3003 = local read "Port for \nC1-Equilibriation"() -> (w3455:string)
                            n3004 = call "PortChanger (SubVI).vi"("Port Number"=w3455, "VISA Refnum in"=w3456) -> ()  [unwired: 10 in]
                          }
                          frame #1 {
                            n3005 = local read "VISA Refnum in\nfor Pump"() -> (w3457:refnum<visa-resource-name>)
                            n3006 = call "ProcessCompletionWaiter (SubVI).vi"("VISA Refnum in"=w3457) -> ()  [unwired: 11 in]
                          }
                          frame #2 {
                            # "Wash the inside of the pump valve"
                            n3007 = local read "n"() -> (w3458:i32)
                            n3008 = for {
                              N: w3458 -> [_]
                              n3009 = stacked-sequence {
                                frame #0 {
                                n3010 = local read "Buffer-A2 Pumping\nResolution"() -> (w3461:T2)
                                n3011 = local read "VISA Refnum in\nfor Pump"() -> (w3463:refnum<visa-resource-name>)
                                n3012 = local read "V-S"() -> (w3459:dbl)
                                n3013 = local read "Volume of Syringe"() -> (w3462:dbl)
                                n3014 = call "RPickUp(SubVI).vi"("Volume to be picked up"=w3459, "Volume of Syringe"=w3462, "Resolution of PickUP"=w3461, "PickUp Flow Rate (ul/min)"=150.0, "VISA Refnum in"=w3463) -> ()  [unwired: 6 in, 1 out]
                                }
                                frame #1 {
                                n3015 = local read "Stopper that ends \nthe main loops"() -> (w3464:bool)
                                n3016 = local read "VISA Refnum in\nfor Pump"() -> (w3465:refnum<visa-resource-name>)
                                n3017 = case shown="True" w3464 {
                                frame False {
                                }
                                frame True {
                                n3018 = local read "VISA Refnum in\nfor Pump"() -> (w3466:refnum<visa-resource-name>)
                                n3019 = call "HardStopCurrentProcess (SubVI).vi"("VISA Refnum in"=w3466) -> ()  [unwired: 11 in]
                                }
                                }
                                n3020 = call "ProcessCompletionWaiter (SubVI).vi"("VISA Refnum in"=w3465) -> ()  [unwired: 11 in]
                                }
                                frame #2 {
                                # "Switch to Port-1"
                                # "Port-1 of the pump is conncted to waste"
                                n3021 = local read "VISA Refnum in\nfor Pump"() -> (w3468:refnum<visa-resource-name>)
                                n3022 = call "PortChanger (SubVI).vi"("Port Number"="1", "VISA Refnum in"=w3468) -> ()  [unwired: 10 in]
                                }
                                frame #3 {
                                n3023 = local read "Stopper that ends \nthe main loops"() -> (w3469:bool)
                                n3024 = local read "VISA Refnum in\nfor Pump"() -> (w3470:refnum<visa-resource-name>)
                                n3025 = case shown="True" w3469 {
                                frame False {
                                }
                                frame True {
                                n3026 = local read "VISA Refnum in\nfor Pump"() -> (w3471:refnum<visa-resource-name>)
                                n3027 = call "HardStopCurrentProcess (SubVI).vi"("VISA Refnum in"=w3471) -> ()  [unwired: 11 in]
                                }
                                }
                                n3028 = call "ProcessCompletionWaiter (SubVI).vi"("VISA Refnum in"=w3470) -> ()  [unwired: 11 in]
                                }
                                frame #4 {
                                n3029 = local read "Buffer-A2 Pumping\nResolution"() -> (w3474:T2)
                                n3030 = local read "VISA Refnum in\nfor Pump"() -> (w3476:refnum<visa-resource-name>)
                                n3031 = local read "Volume of Syringe"() -> (w3475:dbl)
                                n3032 = call "GoToAbsolutePosition(SubVI).vi"("Absolute Volume Position in Syringe (in ul)"=0.0 ("Volume to be Dispensed"), "Volume of Syringe"=w3475, "Resolution of Pumping"=w3474, "Flow Rate (ul/min)"=150.0, "VISA Refnum in"=w3476) -> ()  [unwired: 6 in, 1 out]
                                }
                                frame #5 {
                                n3033 = local read "VISA Refnum in\nfor Pump"() -> (w3477:refnum<visa-resource-name>)
                                n3034 = call "ProcessCompletionWaiter (SubVI).vi"("VISA Refnum in"=w3477) -> ()  [unwired: 11 in]
                                }
                                frame #6 {
                                # "Change the port back to Buffer-C1"
                                n3035 = local read "VISA Refnum in\nfor Pump"() -> (w3479:refnum<visa-resource-name>)
                                n3036 = local read "Port for \nC1-Equilibriation"() -> (w3478:string)
                                n3037 = call "PortChanger (SubVI).vi"("Port Number"=w3478, "VISA Refnum in"=w3479) -> ()  [unwired: 10 in]
                                }
                                frame #7 {
                                n3038 = local read "VISA Refnum in\nfor Pump"() -> (w3480:refnum<visa-resource-name>)
                                n3039 = call "ProcessCompletionWaiter (SubVI).vi"("VISA Refnum in"=w3480) -> ()  [unwired: 11 in]
                                }
                              }
                            }
                          }
                          frame #3 {
                            # "Wash the pathway between column-2 and column-1 on chip"
                            n3040 = local read "n"() -> (w3481:i32)
                            n3041 = for {
                              N: w3481 -> [_]
                              n3042 = stacked-sequence {
                                frame #0 {
                                n3043 = local read "Buffer-A2 Pumping\nResolution"() -> (w3484:T2)
                                n3044 = local read "VISA Refnum in\nfor Pump"() -> (w3486:refnum<visa-resource-name>)
                                n3045 = local read "V-S"() -> (w3482:dbl)
                                n3046 = local read "Volume of Syringe"() -> (w3485:dbl)
                                n3047 = call "RPickUp(SubVI).vi"("Volume to be picked up"=w3482, "Volume of Syringe"=w3485, "Resolution of PickUP"=w3484, "PickUp Flow Rate (ul/min)"=150.0, "VISA Refnum in"=w3486) -> ()  [unwired: 6 in, 1 out]
                                }
                                frame #1 {
                                n3048 = local read "Stopper that ends \nthe main loops"() -> (w3487:bool)
                                n3049 = local read "VISA Refnum in\nfor Pump"() -> (w3488:refnum<visa-resource-name>)
                                n3050 = case shown="True" w3487 {
                                frame False {
                                }
                                frame True {
                                n3051 = local read "VISA Refnum in\nfor Pump"() -> (w3489:refnum<visa-resource-name>)
                                n3052 = call "HardStopCurrentProcess (SubVI).vi"("VISA Refnum in"=w3489) -> ()  [unwired: 11 in]
                                }
                                }
                                n3053 = call "ProcessCompletionWaiter (SubVI).vi"("VISA Refnum in"=w3488) -> ()  [unwired: 11 in]
                                }
                                frame #2 {
                                # "Switch to Port-10"
                                # "Port-10 of the pump is conncted to column-2"
                                n3054 = local read "VISA Refnum in\nfor Pump"() -> (w3491:refnum<visa-resource-name>)
                                n3055 = call "PortChanger (SubVI).vi"("Port Number"="10", "VISA Refnum in"=w3491) -> ()  [unwired: 10 in]
                                }
                                frame #3 {
                                n3056 = local read "Stopper that ends \nthe main loops"() -> (w3492:bool)
                                n3057 = local read "VISA Refnum in\nfor Pump"() -> (w3493:refnum<visa-resource-name>)
                                n3058 = case shown="True" w3492 {
                                frame False {
                                }
                                frame True {
                                n3059 = local read "VISA Refnum in\nfor Pump"() -> (w3494:refnum<visa-resource-name>)
                                n3060 = call "HardStopCurrentProcess (SubVI).vi"("VISA Refnum in"=w3494) -> ()  [unwired: 11 in]
                                }
                                }
                                n3061 = call "ProcessCompletionWaiter (SubVI).vi"("VISA Refnum in"=w3493) -> ()  [unwired: 11 in]
                                }
                                frame #4 {
                                n3062 = local read "Buffer-A2 Pumping\nResolution"() -> (w3503:T2)
                                n3063 = local read "VISA Refnum in\nfor Pump"() -> (w3505:refnum<visa-resource-name>)
                                n3064 = local read "f"() -> (w3495:dbl)
                                n3065 = local read "Volume of Syringe"() -> (w3504:dbl)
                                n3066 = call "GoToAbsolutePosition(SubVI).vi"("Absolute Volume Position in Syringe (in ul)"=0.0 ("Volume to be Dispensed"), "Volume of Syringe"=w3504, "Resolution of Pumping"=w3503, "Flow Rate (ul/min)"=w3495, "VISA Refnum in"=w3505) -> ()  [unwired: 6 in, 1 out]
                                n3067 = local read "VISA Refnum in\nfor Valve"() -> (w3497:refnum<visa-resource-name>)
                                n3068 = local read "External Valve \nOPEN"() -> (w3496:string)
                                n3069 = local write "Valve V2 Open"(TRUE ("Valve V2 Open")) -> ()
                                n3070 = local write "Valve V1 Open"(FALSE ("Valve V1 Open")) -> ()
                                n3071 = local write "Valve V4 Open"(FALSE ("Valve V4 Open")) -> ()
                                n3072 = local write "Valve V3 Open"(TRUE ("Valve V3 Open")) -> ()
                                n3073 = call "PortChanger_Valve (SubVI).vi"("Port Number"=w3496, "VISA Refnum in"=w3497) -> ()  [unwired: 10 in]
                                }
                                frame #5 {
                                n3074 = local read "VISA Refnum in\nfor Pump"() -> (w3506:refnum<visa-resource-name>)
                                n3075 = call "ProcessCompletionWaiter (SubVI).vi"("VISA Refnum in"=w3506) -> ()  [unwired: 11 in]
                                }
                                frame #6 {
                                # "Change the port back to Buffer-C1"
                                n3076 = local read "VISA Refnum in\nfor Pump"() -> (w3508:refnum<visa-resource-name>)
                                n3077 = local read "Port for \nC1-Equilibriation"() -> (w3507:string)
                                n3078 = call "PortChanger (SubVI).vi"("Port Number"=w3507, "VISA Refnum in"=w3508) -> ()  [unwired: 10 in]
                                }
                                frame #7 {
                                n3079 = local read "VISA Refnum in\nfor Pump"() -> (w3509:refnum<visa-resource-name>)
                                n3080 = call "ProcessCompletionWaiter (SubVI).vi"("VISA Refnum in"=w3509) -> ()  [unwired: 11 in]
                                }
                              }
                            }
                          }
                          frame #4 {
                            # "Washes the SEC column"
                            n3081 = local read "Apparent Volume\nof Syringe"() -> (w3512:dbl)
                            n3082 = local read "c"() -> (w3513:dbl)
                            n3083 = Quotient & Remainder(x=w3513, y=w3512) -> (x-y*floor(x/y)=w3511:dbl, floor(x/y)=w3510:dbl)
                            n3084 = for {
                              N: w3510 -> [_]
                              n3085 = stacked-sequence {
                                frame #0 {
                                n3086 = local read "Buffer-A2 Pumping\nResolution"() -> (w3516:T2)
                                n3087 = local read "VISA Refnum in\nfor Pump"() -> (w3518:refnum<visa-resource-name>)
                                n3088 = local read "Apparent Volume\nof Syringe"() -> (w3514:dbl)
                                n3089 = local read "Volume of Syringe"() -> (w3517:dbl)
                                n3090 = call "RPickUp(SubVI).vi"("Volume to be picked up"=w3514, "Volume of Syringe"=w3517, "Resolution of PickUP"=w3516, "PickUp Flow Rate (ul/min)"=150.0, "VISA Refnum in"=w3518) -> ()  [unwired: 6 in, 1 out]
                                }
                                frame #1 {
                                n3091 = local read "Stopper that ends \nthe main loops"() -> (w3519:bool)
                                n3092 = local read "VISA Refnum in\nfor Pump"() -> (w3520:refnum<visa-resource-name>)
                                n3093 = case shown="True" w3519 {
                                frame False {
                                }
                                frame True {
                                n3094 = local read "VISA Refnum in\nfor Pump"() -> (w3521:refnum<visa-resource-name>)
                                n3095 = call "HardStopCurrentProcess (SubVI).vi"("VISA Refnum in"=w3521) -> ()  [unwired: 11 in]
                                }
                                }
                                n3096 = call "ProcessCompletionWaiter (SubVI).vi"("VISA Refnum in"=w3520) -> ()  [unwired: 11 in]
                                }
                                frame #2 {
                                # "Switch to Port-10"
                                # "Port-10 of the pump is conncted to column-2 of chip"
                                n3097 = local read "VISA Refnum in\nfor Pump"() -> (w3523:refnum<visa-resource-name>)
                                n3098 = call "PortChanger (SubVI).vi"("Port Number"="10", "VISA Refnum in"=w3523) -> ()  [unwired: 10 in]
                                }
                                frame #3 {
                                n3099 = local read "Stopper that ends \nthe main loops"() -> (w3524:bool)
                                n3100 = local read "VISA Refnum in\nfor Pump"() -> (w3525:refnum<visa-resource-name>)
                                n3101 = case shown="True" w3524 {
                                frame False {
                                }
                                frame True {
                                n3102 = local read "VISA Refnum in\nfor Pump"() -> (w3526:refnum<visa-resource-name>)
                                n3103 = call "HardStopCurrentProcess (SubVI).vi"("VISA Refnum in"=w3526) -> ()  [unwired: 11 in]
                                }
                                }
                                n3104 = call "ProcessCompletionWaiter (SubVI).vi"("VISA Refnum in"=w3525) -> ()  [unwired: 11 in]
                                }
                                frame #4 {
                                # "Keeps the AMF valve after column-1 open and valve after column-2 closed"
                                n3105 = local read "Buffer-A2 Pumping\nResolution"() -> (w3538:T2)
                                n3106 = local read "VISA Refnum in\nfor Pump"() -> (w3540:refnum<visa-resource-name>)
                                n3107 = local read "f"() -> (w3530:dbl)
                                n3108 = local write "Valve V3 Open"(FALSE ("Valve V3 Open")) -> ()
                                n3109 = local write "Valve V2 Open"(FALSE ("Valve V2 Open")) -> ()
                                n3110 = local write "Valve V4 Open"(TRUE ("Valve V4 Open")) -> ()
                                n3111 = local write "Valve V1 Open"(FALSE ("Valve V1 Open")) -> ()
                                n3112 = local read "Volume of Syringe"() -> (w3539:dbl)
                                n3113 = call "GoToAbsolutePosition(SubVI).vi"("Absolute Volume Position in Syringe (in ul)"=0.0 ("Volume to be Dispensed"), "Volume of Syringe"=w3539, "Resolution of Pumping"=w3538, "Flow Rate (ul/min)"=w3530, "VISA Refnum in"=w3540) -> ()  [unwired: 6 in, 1 out]
                                n3114 = local read "VISA Refnum in\nfor Valve"() -> (w3535:refnum<visa-resource-name>)
                                n3115 = local read "External Valve \nCLOSED"() -> (w3531:string)
                                n3116 = local write "Valve V5 Open"(TRUE ("Valve V5 Open")) -> ()
                                n3117 = local write "Valve V6 Open"(FALSE ("Valve V6 Open")) -> ()
                                n3118 = local write "Valve V7 Open"(TRUE ("Valve V7 Open")) -> ()
                                n3119 = call "PortChanger_Valve (SubVI).vi"("Port Number"=w3531, "VISA Refnum in"=w3535) -> ()  [unwired: 10 in]
                                }
                                frame #5 {
                                n3120 = local read "VISA Refnum in\nfor Pump"() -> (w3541:refnum<visa-resource-name>)
                                n3121 = call "ProcessCompletionWaiter (SubVI).vi"("VISA Refnum in"=w3541) -> ()  [unwired: 11 in]
                                }
                                frame #6 {
                                # "Change the port back to Buffer-C1"
                                n3122 = local read "VISA Refnum in\nfor Pump"() -> (w3543:refnum<visa-resource-name>)
                                n3123 = local read "Port for \nC1-Equilibriation"() -> (w3542:string)
                                n3124 = call "PortChanger (SubVI).vi"("Port Number"=w3542, "VISA Refnum in"=w3543) -> ()  [unwired: 10 in]
                                }
                                frame #7 {
                                n3125 = local read "VISA Refnum in\nfor Pump"() -> (w3544:refnum<visa-resource-name>)
                                n3126 = call "ProcessCompletionWaiter (SubVI).vi"("VISA Refnum in"=w3544) -> ()  [unwired: 11 in]
                                }
                              }
                            }
                            n3127 = local write "Reminder of the \nVolume to be \nPumped"(w3511) -> ()
                          }
                          frame #5 {
                            # "Washes the SEC column"
                            n3128 = stacked-sequence {
                              frame #0 {
                                n3129 = local read "Buffer-A2 Pumping\nResolution"() -> (w3547:T2)
                                n3130 = local read "VISA Refnum in\nfor Pump"() -> (w3549:refnum<visa-resource-name>)
                                n3131 = local read "Reminder of the \nVolume to be \nPumped"() -> (w3545:dbl)
                                n3132 = local read "Volume of Syringe"() -> (w3548:dbl)
                                n3133 = call "RPickUp(SubVI).vi"("Volume to be picked up"=w3545, "Volume of Syringe"=w3548, "Resolution of PickUP"=w3547, "PickUp Flow Rate (ul/min)"=150.0, "VISA Refnum in"=w3549) -> ()  [unwired: 6 in, 1 out]
                              }
                              frame #1 {
                                n3134 = local read "Stopper that ends \nthe main loops"() -> (w3550:bool)
                                n3135 = local read "VISA Refnum in\nfor Pump"() -> (w3551:refnum<visa-resource-name>)
                                n3136 = case shown="True" w3550 {
                                frame False {
                                }
                                frame True {
                                n3137 = local read "VISA Refnum in\nfor Pump"() -> (w3552:refnum<visa-resource-name>)
                                n3138 = call "HardStopCurrentProcess (SubVI).vi"("VISA Refnum in"=w3552) -> ()  [unwired: 11 in]
                                }
                                }
                                n3139 = call "ProcessCompletionWaiter (SubVI).vi"("VISA Refnum in"=w3551) -> ()  [unwired: 11 in]
                              }
                              frame #2 {
                                # "Switch to Port-10"
                                # "Port-10 of the pump is conncted to column-2 of chip"
                                n3140 = local read "VISA Refnum in\nfor Pump"() -> (w3554:refnum<visa-resource-name>)
                                n3141 = call "PortChanger (SubVI).vi"("Port Number"="10", "VISA Refnum in"=w3554) -> ()  [unwired: 10 in]
                              }
                              frame #3 {
                                n3142 = local read "Stopper that ends \nthe main loops"() -> (w3555:bool)
                                n3143 = local read "VISA Refnum in\nfor Pump"() -> (w3556:refnum<visa-resource-name>)
                                n3144 = case shown="True" w3555 {
                                frame False {
                                }
                                frame True {
                                n3145 = local read "VISA Refnum in\nfor Pump"() -> (w3557:refnum<visa-resource-name>)
                                n3146 = call "HardStopCurrentProcess (SubVI).vi"("VISA Refnum in"=w3557) -> ()  [unwired: 11 in]
                                }
                                }
                                n3147 = call "ProcessCompletionWaiter (SubVI).vi"("VISA Refnum in"=w3556) -> ()  [unwired: 11 in]
                              }
                              frame #4 {
                                n3148 = local read "Buffer-A2 Pumping\nResolution"() -> (w3569:T2)
                                n3149 = local read "VISA Refnum in\nfor Pump"() -> (w3571:refnum<visa-resource-name>)
                                n3150 = local read "f"() -> (w3561:dbl)
                                n3151 = local read "Volume of Syringe"() -> (w3570:dbl)
                                n3152 = call "GoToAbsolutePosition(SubVI).vi"("Absolute Volume Position in Syringe (in ul)"=0.0 ("Volume to be Dispensed"), "Volume of Syringe"=w3570, "Resolution of Pumping"=w3569, "Flow Rate (ul/min)"=w3561, "VISA Refnum in"=w3571) -> ()  [unwired: 6 in, 1 out]
                                n3153 = local write "Valve V3 Open"(FALSE ("Valve V3 Open")) -> ()
                                n3154 = local write "Valve V2 Open"(FALSE ("Valve V2 Open")) -> ()
                                n3155 = local write "Valve V1 Open"(FALSE ("Valve V1 Open")) -> ()
                                n3156 = local write "Valve V4 Open"(TRUE ("Valve V4 Open")) -> ()
                                n3157 = local read "VISA Refnum in\nfor Valve"() -> (w3566:refnum<visa-resource-name>)
                                n3158 = local read "External Valve \nCLOSED"() -> (w3562:string)
                                n3159 = local write "Valve V6 Open"(TRUE ("Valve V6 Open")) -> ()
                                n3160 = local write "Valve V5 Open"(TRUE ("Valve V5 Open")) -> ()
                                n3161 = local write "Valve V7 Open"(TRUE ("Valve V7 Open")) -> ()
                                n3162 = call "PortChanger_Valve (SubVI).vi"("Port Number"=w3562, "VISA Refnum in"=w3566) -> ()  [unwired: 10 in]
                              }
                              frame #5 {
                                n3163 = local read "VISA Refnum in\nfor Pump"() -> (w3572:refnum<visa-resource-name>)
                                n3164 = call "ProcessCompletionWaiter (SubVI).vi"("VISA Refnum in"=w3572) -> ()  [unwired: 11 in]
                              }
                            }
                          }
                        }
                        n3165 = local write "Washing Column-1"(FALSE ("Washing Column-1")) -> ()
                        n3166 = local write "Washing Column-2"(TRUE ("Washing Column-2")) -> ()
                      }
                      frame #4 {
                        # "Elute Column-1, Divert Sample into Column-2, Elute column-2 and Divert the sample onto Grid"
                        n3167 = stacked-sequence {
                          frame #0 {
                            # "Switch to Port-7"
                            # "Port-7 of pump is connected to Buffer-B"
                            n3168 = local write "Washing Column-2"(FALSE ("Washing Column-2")) -> ()
                            n3169 = local read "VISA Refnum in\nfor Pump"() -> (w3577:refnum<visa-resource-name>)
                            n3170 = local read "Port for \nB-Elution"() -> (w3575:string)
                            n3171 = local write "Affinity Elution On"(TRUE ("Affinity Elution On")) -> ()
                            n3172 = call "PortChanger (SubVI).vi"("Port Number"=w3575, "VISA Refnum in"=w3577) -> ()  [unwired: 10 in]
                            n3173 = local write "Elution of Column-1"(TRUE ("Elution of Column-1")) -> ()
                          }
                          frame #1 {
